vi "Team Data Control.vi"(9 "GUID To Modify":u16, 10 "Team Data To Add/Change":T1, 11 "Mode":T2(ring)) -> (2 "Team Array Out":T1[](array[typedef]))   [LabVIEW 2013]
uses:
  Team Data.ctl
  Team Data Array.ctl
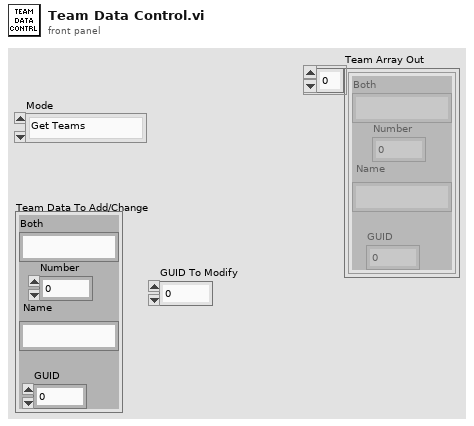
[diagram p1: front panel]
types:
  T1 = typedef "Team Data.ctl" = cluster{"Both":string, "Name":string, "GUID":u16, "Number":u16}
  T2 = enum16{"Get Teams", "Add Team", "Modify Team", "Clear All Teams", "Force Add Team", "Delete Team", "Add Team With GUID"}
  T3 = typedef "Team Data Array.ctl" = T1[]
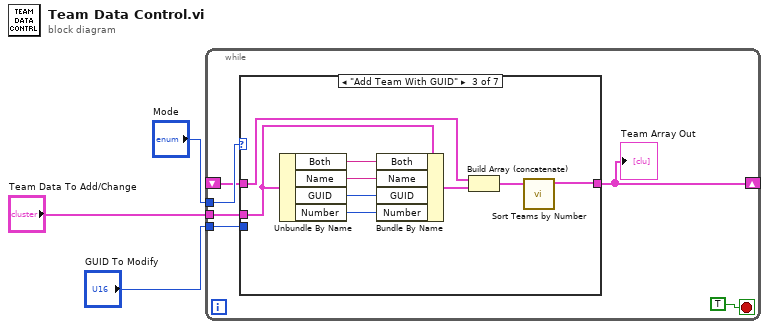
[diagram p0: block diagram]
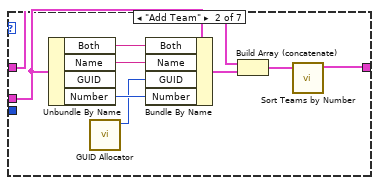
[diagram p3: hidden frame]
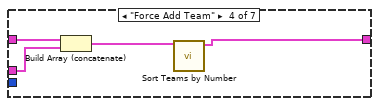
[diagram p4: hidden frame]
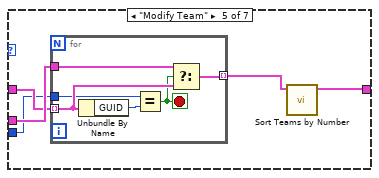
[diagram p5: hidden frame]
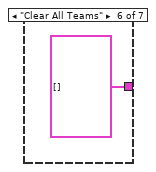
[diagram p6: hidden frame]
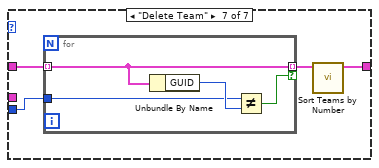
[diagram p7: hidden frame]
diagram:
  n1 = while {
    tunnel: "Mode" -> [w9]
    tunnel: "Team Data To Add/Change" -> [w8]
    tunnel: "GUID To Modify" -> [w7]
    shift-right: [w6] -> _
    shift-left: _ -> [w5]
    stop <- TRUE stop-if-true
    n2 = case shown="\"Add Team With GUID\"" w9 {
      tunnel: w5 -> [w10 w19 w28 w32 w36 _ w48]
      tunnel: [w10 w11 w21 w29 w34 T3 [] ("Team Info") w45] -> w6
      tunnel: w8 -> [_ w13 w23 w31 w37 _ _]
      tunnel: w7 -> [_ _ _ _ w35 _ w47]
      frame "Get Teams", Default {
      }
      frame "Add Team" {
        n3 = Unbundle By Name(w13) -> ("Both"=w18:string, "Name"=w17:string, "Number"=w16:u16)  [unwired: 1 out]
        n4 = call "GUID Allocator.vi"() -> ("New GUID"=w15:u16)  [unwired: 11 in]
        n5 = Bundle By Name(cluster=w13, "Both"=w18, "Name"=w17, "GUID"=w15, "Number"=w16) -> (w14:T1)
        n6 = Build Array (concatenate)(w19, w14) -> (w12:T3)
        n7 = call "Sort Teams by Number.vi"("Team Info"=w12) -> ("Array"=w11:T1[])  [unwired: 10 in]
      }
      frame "Add Team With GUID" {
        n8 = Unbundle By Name(w23) -> ("Both"=w27:string, "Name"=w26:string, "GUID"=w20:u16, "Number"=w25:u16)
        n9 = Bundle By Name(cluster=w23, "Both"=w27, "Name"=w26, "GUID"=w20, "Number"=w25) -> (w24:T1)
        n10 = Build Array (concatenate)(w28, w24) -> (w22:T3)
        n11 = call "Sort Teams by Number.vi"("Team Info"=w22) -> ("Array"=w21:T1[])  [unwired: 10 in]
      }
      frame "Force Add Team" {
        n12 = Build Array (concatenate)(w32, w31) -> (w30:T3)
        n13 = call "Sort Teams by Number.vi"("Team Info"=w30) -> ("Array"=w29:T1[])  [unwired: 10 in]
      }
      frame "Modify Team" {
        n14 = for {
          tunnel: w36 -> [w41] mode=indexing
          tunnel: [w43] -> w33 mode=indexing
          tunnel: w37 -> [w42]
          tunnel: w35 -> [w39]
          stop <- w38 stop-if-true
          n15 = Unbundle By Name(w41) -> ("GUID"=w40:u16)
          n16 = Equal?(x=w39, y=w40) -> (x = y?=w38:bool)
          n17 = Select(t=w42, s=w38, f=w41) -> (s? t:f=w43:T1)
        }
        n18 = call "Sort Teams by Number.vi"("Team Info"=w33) -> ("Array"=w34:T1[])  [unwired: 10 in]
      }
      frame "Clear All Teams" {
      }
      frame "Delete Team" {
        n19 = for {
          tunnel: w48 -> [w50] mode=indexing
          tunnel: w47 -> [w51]
          tunnel: [w50] -> w46 mode=indexing if=w49
          n20 = Unbundle By Name(w50) -> ("GUID"=w52:u16)
          n21 = Not Equal?(x=w51, y=w52) -> (x != y?=w49:bool)
        }
        n22 = call "Sort Teams by Number.vi"("Team Info"=w46) -> ("Array"=w45:T1[])  [unwired: 10 in]
      }
    }
    "Team Array Out" <- w6
  }
